vi "Python_node_benchmarking.vi"() -> ()   [LabVIEW 2018]
uses:
  <vilib>/Utility/file.llb/Read Delimited Spreadsheet (DBL).vi
panel:
  out "time for loop":dbl
  in  "stop":bool
  out "time":dbl
  in  "Output type":sgl[][](array[numeric])
  out "all rows 2":dbl[][](array[numeric])
  out "output + time from code":dbl[][](array[numeric])
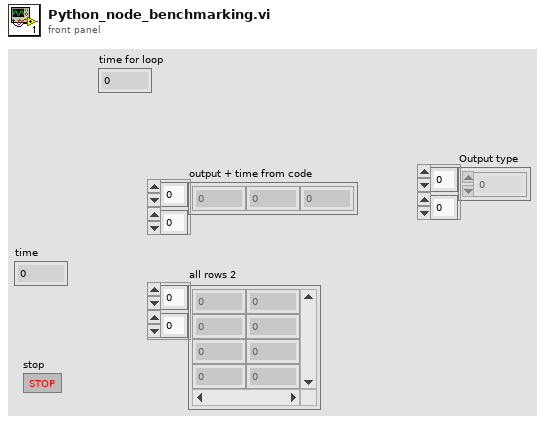
[diagram p1: front panel]
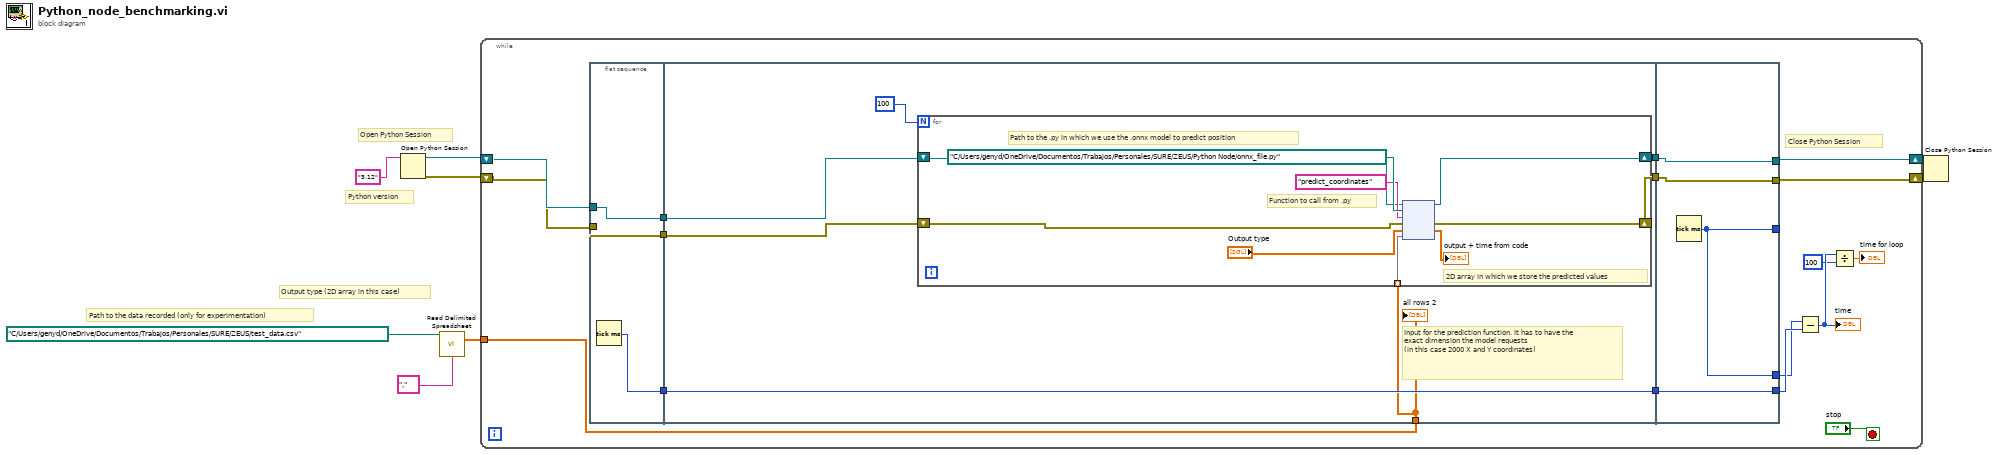
[diagram p0: block diagram]
diagram:
  # "Open Python Session"
  # "Output type (2D array in this case)"
  # "Path to the data recorded (only for experimentation)"
  # "Python version"
  n1 = Open Python Session(python version="3.12" ("Python version")) -> (session out=w7:refnum<k35>, error out=w6:errorcluster)  [unwired: 2 in]
  n2 = call-poly <vilib>:"Read Delimited Spreadsheet.vi"("file path (dialog if empty)"=path "C:/Users/genyd/OneDrive/Documentos/Trabajos/Personales/SURE/ZEUS/test_data.csv", "delimiter (\\t)"="," ("delimiter (\\t)")) -> ("all rows"=w1:dbl[][])  [unwired: 8 in, 5 out]
  n3 = while {
    tunnel: w1 -> [w15]
    shift-right: [w17] -> w5
    shift-left: w7 -> [w19]
    shift-right: [w16] -> w4
    shift-left: w6 -> [w18]
    stop <- "stop" stop-if-true
    # "Close Python Session"
    n4 = flat-sequence {
      tunnel: [w28] -> w25
      tunnel: [w27] -> w24
      tunnel: w19 -> [w28]
      tunnel: w18 -> [w27]
      tunnel: [w26] -> w23
      tunnel: w25 -> [w35]
      tunnel: w24 -> [w34]
      tunnel: [w33] -> w22
      tunnel: [w32] -> w21
      tunnel: [w31] -> w20
      tunnel: w23 -> [w31]
      tunnel: w15 -> [w30]
      tunnel: [w45] -> w13
      tunnel: w22 -> [w48]
      tunnel: w21 -> [w47]
      tunnel: [w48] -> w17
      tunnel: [w47] -> w16
      tunnel: [w46] -> w14
      tunnel: w20 -> [w46]
      tunnel: [w45] -> _
      frame #0 {
        n5 = Tick Count (ms)() -> (millisecond timer value=w26:u32)
      }
      frame #1 {
        # "Input for the prediction function. It has to have the exact dimension the model requests \n(in this case 2000 X and Y coordinates)"
        n6 = for {
          N: 100 -> [_]
          tunnel: w30 -> [w36] mode=indexing
          shift-right: [w38] -> w33
          shift-left: w35 -> [w40]
          shift-right: [w37] -> w32
          shift-left: w34 -> [w39]
          # "2D array in which we store the predicted values"
          # "Function to call from .py"
          # "Path to the .py in which we use the .onnx model to predict position"
          n7 = node(w40, path "C:/Users/genyd/OneDrive/Documentos/Trabajos/Personales/SURE/ZEUS/Python Node/onnx_file.py" ("module path"), "predict_coordinates" ("function name"), w39, "Output type", w36) -> (w38:refnum<k35>, w37:errorcluster, →"output + time from code":sgl[][])  [unwired: 1 in, 2 out]
        }
        "all rows 2" <- w30
      }
      frame #2 {
        n8 = Tick Count (ms)() -> (millisecond timer value=w45:u32)
      }
    }
    n9 = Subtract(x=w13, y=w14) -> (x-y=w11:u32)
    "time" <- w11
    n10 = Divide(x=w11, y=u32 100) -> (x/y=→"time for loop":dbl)
  }
  n11 = Close Python Session(session in=w5, error in=w4) -> ()  [unwired: 1 out]
